vi "Fetch Trace (Swept SA) (bytes override).vi"(0 "VISA resource name":refnum<visa-resource-name>, 5 "Timeout (10000 ms)":i32=10000 format="%.0g", 7 "byte count":u32=100000, 9 "Trace Name (1: Trace 1)":i32(ring)=1 items=["Trace 1"=1, "Trace 2"=2, "Trace 3"=3, "Trace 4"=4, "Trace 5"=5, "Trace 6"=6], 11 "error in (no error)":errorcluster) -> (4 "VISA resource name out":refnum<visa-resource-name>, 6 "X Array":dbl[](array[numeric]), 10 "Y Array":dbl[](array[numeric]), 15 "error out":errorcluster)   [LabVIEW 2014]
doc: "Fetches trace from the spectrum analyzer (Swept SA) and does not initiate data acquisition.\n\n<B>Note:</B>\n\nUse this VI only with other low-level VIs. The high-level VIs automatically incorporate this functionality. This VI does not check the instrument status."
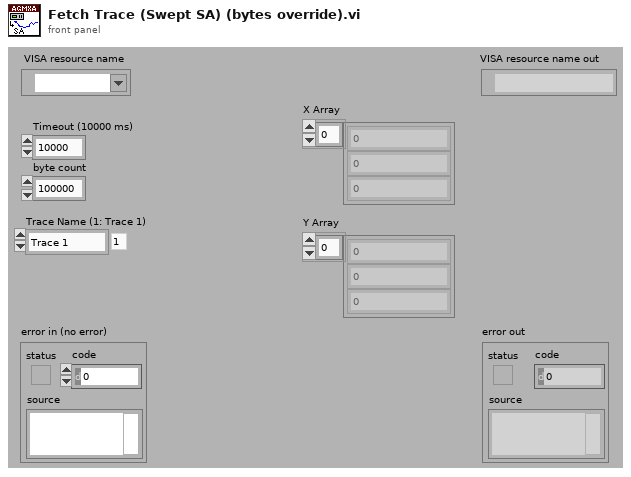
[diagram p1: front panel]
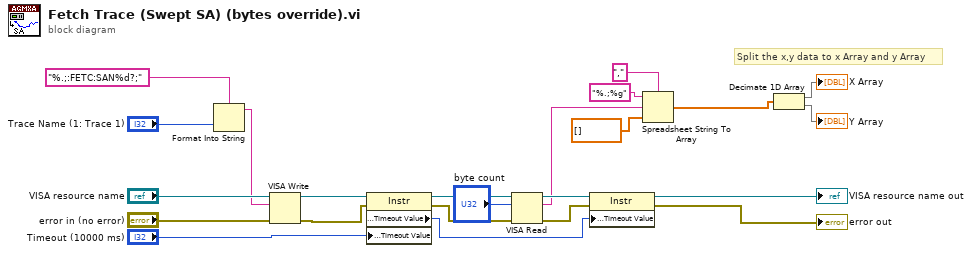
[diagram p0: block diagram]
diagram:
  # "Split the x,y data to x Array and y Array"
  n1 = Format Into String(format string="%.;:FETC:SAN%d?;", "Trace Name (1: Trace 1)") -> (resulting string=w17:string)  [unwired: 2 in, 1 out]
  n2 = VISA Write(VISA resource name="VISA resource name", write buffer=w17, error in (no error)="error in (no error)") -> (VISA resource name out=w19:refnum<visa-resource-name>, error out=w3:errorcluster)  [unwired: 1 out]
  n3 = property on="Property Node" class="Instr"(reference=w19, error in=w3, "General Settings:Timeout Value"="Timeout (10000 ms)") -> (reference out=w13:refnum<visa-resource-name>, error out=w2:errorcluster, "General Settings:Timeout Value"=w9:u32)
  n4 = VISA Read(VISA resource name=w13, byte count="byte count", error in (no error)=w2) -> (VISA resource name out=w12:refnum<visa-resource-name>, read buffer=w11:string, error out=w10:errorcluster)  [unwired: 1 out]
  n5 = property on="Property Node" class="Instr"(reference=w12, error in=w10, "General Settings:Timeout Value"=w9) -> (reference out=→"VISA resource name out":refnum<visa-resource-name>, error out=→"error out":errorcluster)
  n6 = Spreadsheet String To Array(delimiter (Tab)=",", format string="%.;%g", spreadsheet string=w11, array type (2D Dbl)=dbl[] []) -> (array=w6:dbl[])
  n7 = Decimate 1D Array(w6) -> (→"X Array":dbl[], →"Y Array":dbl[])
